vi "Find Row Reflection of With Smudge.vi"(11 "2D array":bool[][](array[boolean])) -> (2 "Reflection found":bool, 3 "Row index of reflection":i32)   [LabVIEW 2023]
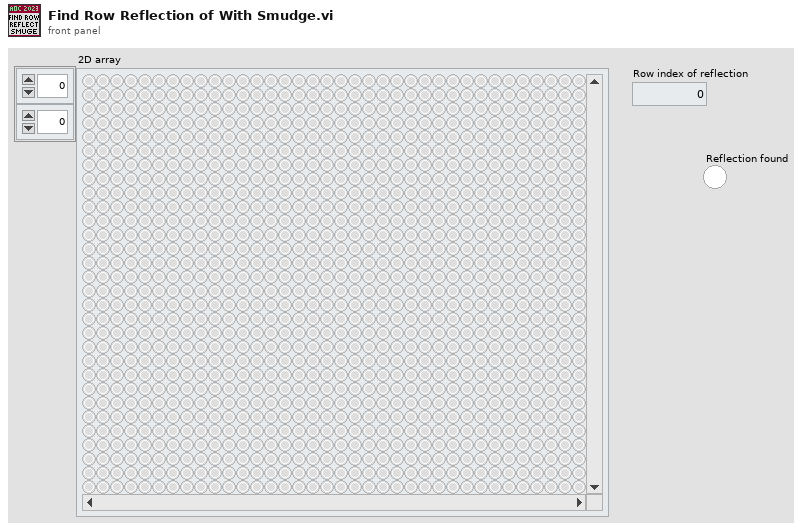
[diagram p1: front panel]
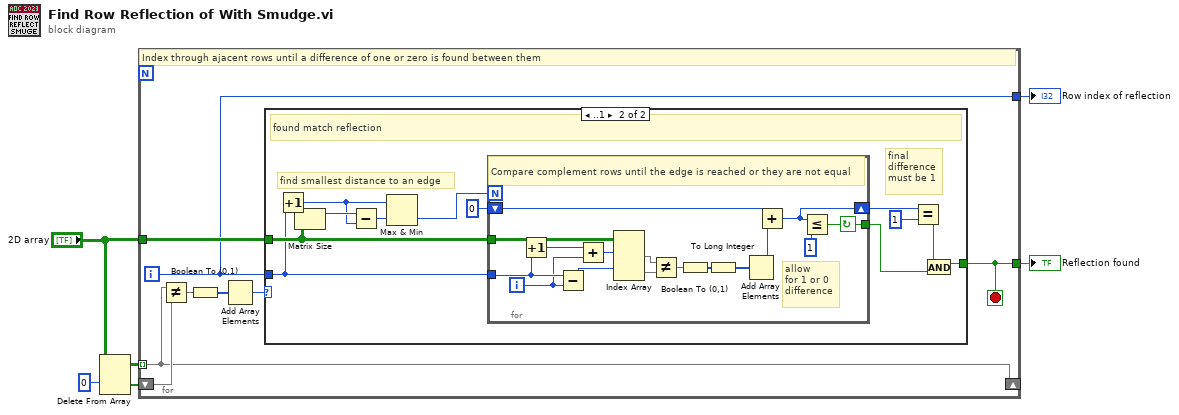
[diagram p0: block diagram]
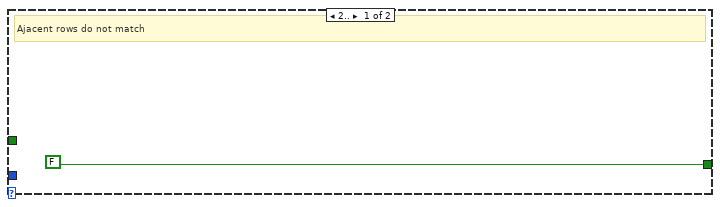
[diagram p2: hidden frame]
diagram:
  n1 = Delete From Array(array="2D array", index (row)=0) -> (deleted portion=w2:bool[], array with subset deleted=w3:bool[][])  [unwired: 2 in]
  n2 = for {
    shift-right: [w13] -> _
    shift-left: w2 -> [w14]
    tunnel: w3 -> [w13] mode=indexing
    tunnel: "2D array" -> [w12]
    tunnel: [w11] -> w5
    tunnel: [w10] -> w6
    i -> [w10]
    stop <- w11 stop-if-true
    # "Index through ajacent rows until a difference of one or zero is found between them"
    n3 = Not Equal?(x=w13, y=w14) -> (x != y?=w9:bool[])
    n4 = Boolean To (0,1)(Boolean=w9) -> (0, 1=w8:i16[])
    n5 = Add Array Elements(numeric array=w8) -> (sum=w7:i16)
    n6 = case shown="..1" w7 {
      tunnel: w12 -> [_ w27]
      tunnel: w10 -> [_ w25]
      tunnel: [FALSE w18] -> w11
      frame 2.. {
        # "Ajacent rows do not match"
      }
      frame ..1 {
        # "final \ndifference\nmust be 1"
        # "find smallest distance to an edge"
        # "found match reflection"
        n7 = Increment(x=w25) -> (x+1=w16:i32)
        n8 = Matrix Size(0:w27) -> (1:w26:i32)  [unwired: 1 out]
        n9 = Subtract(x=w26, y=w16) -> (x-y=w24:i32)
        n10 = Max & Min(x=w16, y=w24) -> (min(x,y)=w23:i32)  [unwired: 1 out]
        n11 = for {
          N: w23 -> [_]
          tunnel: w27 -> [w40]
          tunnel: w25 -> [w43]
          shift-right: [w29] -> w21
          shift-left: 0 -> [w33]
          tunnel: [w28] -> w17
          i -> [w41]
          stop <- w28 continue-if-true
          # "allow\nfor 1 or 0\ndifference"
          # "Compare complement rows until the edge is reached or they are not equal"
          n12 = Increment(x=w43) -> (x+1=w42:i32)
          n13 = Subtract(x=w43, y=w41) -> (x-y=w38:i32)
          n14 = Add(x=w42, y=w41) -> (x+y=w39:i32)
          n15 = Index Array(array=w40, index (row) #1=w39, index (row) #2=w38) -> (element #1=w35:bool[], element #2=w34:bool[])  [unwired: 2 in]
          n16 = Not Equal?(x=w35, y=w34) -> (x != y?=w37:bool[])
          n17 = Boolean To (0,1)(Boolean=w37) -> (0, 1=w36:i16[])
          n18 = To Long Integer(number=w36) -> (32bit integer=w31:i32[])
          n19 = Add Array Elements(numeric array=w31) -> (sum=w32:i32)
          n20 = Add(x=w33, y=w32) -> (x+y=w29:i32)
          n21 = Less Or Equal?(x=w29, y=1) -> (x <= y?=w28:bool)
        }
        n22 = Equal?(x=w21, y=1) -> (x = y?=w19:bool)
        n23 = And(x=w19, y=w17) -> (x .and. y?=w18:bool)
      }
    }
  }
  "Row index of reflection" <- w6
  "Reflection found" <- w5
